vi "Resisitivity of 6-Contact Sample Test.vi"(8 "error in (no error)":errorcluster) -> (0 "error out":errorcluster)   [LabVIEW 2016, in "Hall Effect Library.lvlib"]
doc: "This VI executes the Van Der Pauw Resisitivty Test and returns the voltage measurements V1-V8 taken during the test."
uses:
  Hall Effect Library.lvlib
  Controls/Measurement.ctl
  Public/Controls/Data Items.ctl
  Public/Controls/Tests.ctl
  Global Variables/Test Settings.vi
  Global Variables/Instrument Locations.vi
  Global Variables/Hall Effect Data.vi
panel:
  out "Soak Until":timestamp
  out "Measurement":T1
  out "Test Step":T2(ring)
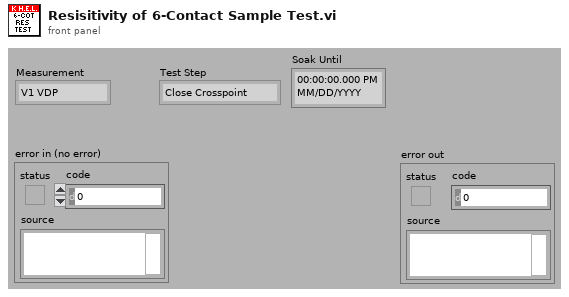
[diagram p1: front panel]
types:
  T1 = typedef "Hall Effect Library.lvlib/Measurement.ctl" = enum16{"V1 VDP", "V2 VDP", "V3 VDP", "V4 VDP", "V5 VDP", "V6 VDP", "V7 VDP", "V8 VDP", "V1 HE", "V2 HE", "V3 HE", "V4 HE", "V5 HE", "V6 HE", "V7 HE", "V8 HE", "V1 Res Bar", "V1 Hall Bar", "V1 Res 6-Cot", "V2 Res 6-Cot", "V3 Res 6-Cot", "V4 Res 6-Cot", "V1 Hall 6-Cot", "V2 Hall 6-Cot", "V3 Hall 6-Cot", "V4 Hall 6-Cot", "V5 Hall 6-Cot", "V6 Hall 6-Cot", "V7 Hall 6-Cot", "V8 Hall 6-Cot", "V1 Res 8-Cot", "V2 Res 8-Cot", "V3 Res 8-Cot", "V4 Res 8-Cot", "V1 Hall 8-Cot", "V2 Hall 8-Cot", "V3 Hall 8-Cot", "V4 Hall 8-Cot"}
  T2 = enum16{"Close Crosspoint", "Soak 1", "Zero Ammeter", "Zero Voltmeter", "I-SRC On", "Init Ammeter", "Soak 2", "Measure I", "Measure V", "I-SRC Off", "Open Crosspoint", "Done"}
  T3 = typedef "Hall Effect Library.lvlib/Resisitivity.ctl" = enum16{"Low", "High"}
  T4 = typedef "Hall Effect Library.lvlib/Tests.ctl" = enum16{"Van Der Pauw", "Hall Effect", "Bar Sample Resistivity", "Bar Sample Hall ", "6-Contact Sample Resistivity", "6-Contact Sample Hall", "8-Contact Sample Resistivity", "8-Contact Sample Hall", ""}
  T5 = typedef "Hall Effect Library.lvlib/Data Items.ctl" = enum16{"V1 Van Der Pauw", "V2 Van Der Pauw", "V3 Van Der Pauw", "V4 Van Der Pauw", "V5 Van Der Pauw", "V6 Van Der Pauw", "V7 Van Der Pauw", "V8 Van Der Pauw", "V1 Hall Effect", "V2 Hall Effect", "V3 Hall Effect", "V4 Hall Effect", "V5 Hall Effect", "V6  Hall Effect", "V7 Hall Effect", "V8 Hall Effect", "V1 Res Bar", "V1 Hall Bar", "V1 Res 6-Cot", "V2 Res 6-Cot", "V3 Res 6-Cot", "V4 Res 6-Cot", "V1 Hall 6-Cot", "V2 Hall 6-Cot", "V3 Hall 6-Cot", "V4 Hall 6-Cot", "V5 Hall 6-Cot", "V6 Hall 6-Cot", "V7 Hall 6-Cot", "V8 Hall 6-Cot", "V1 Res 8-Cot", "V2 Res 8-Cot", "V3 Res 8-Cot", "V4 Res 8-Cot", "V1 Hall 8-Cot", "V2 Hall 8-Cot", "V3 Hall 8-Cot", "V4 Hall 8-Cot", "Van Der Pauw Results", "Hall Effect Results", "Bar Sample Resistivity Results", "Bar Sample Hall Results", "6-Contact Resistivity Results", "6-Contact Hall Results", "8-Contact Resistivity Results", "8-Contact Hall Results"}
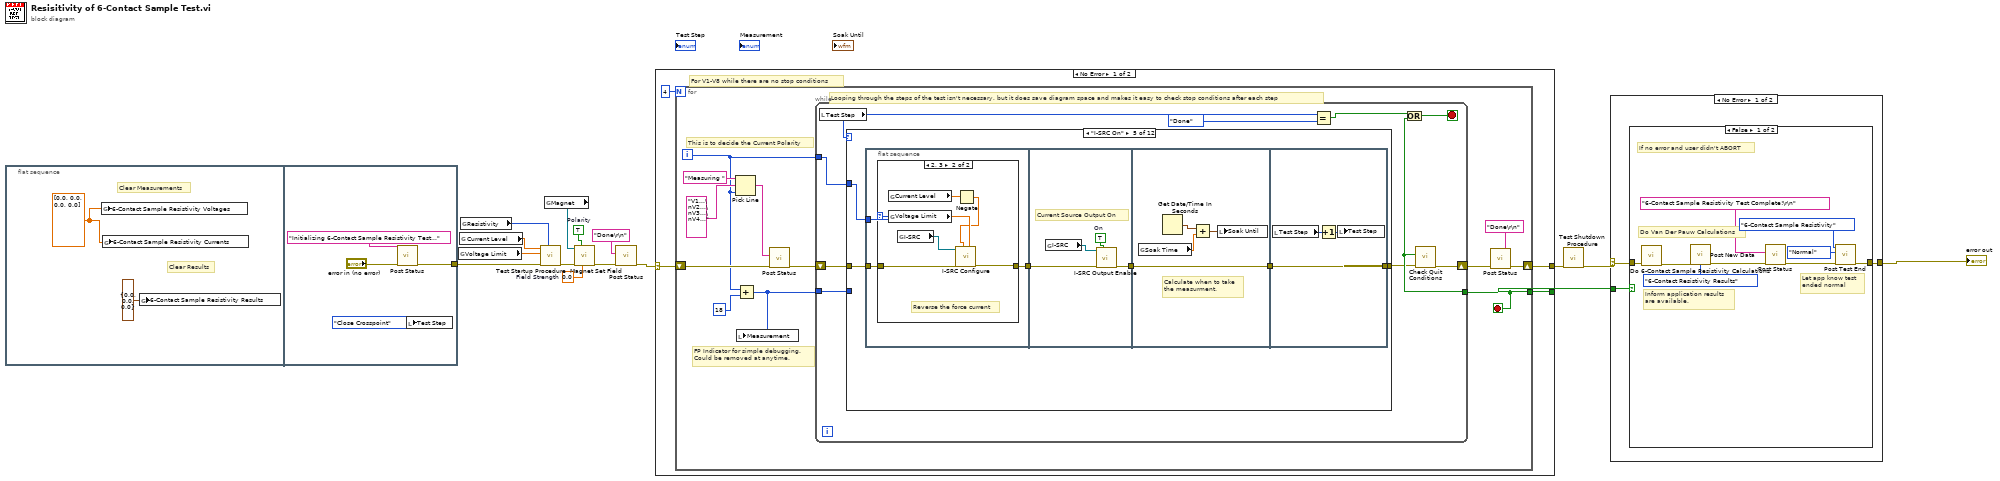
[diagram p0: block diagram]
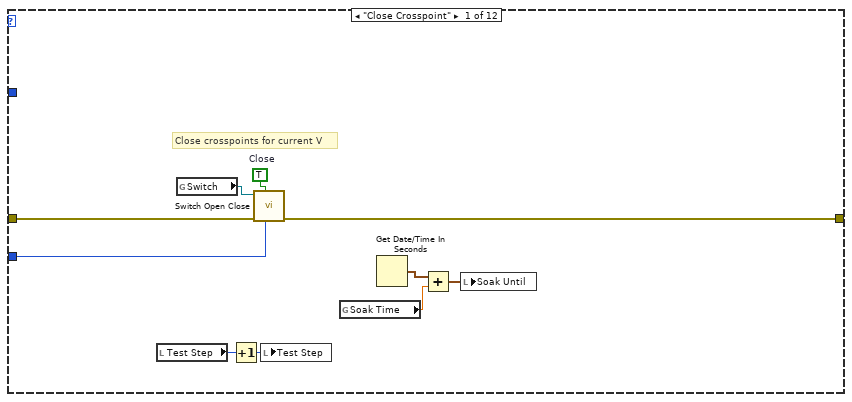
[diagram p2: hidden frame]
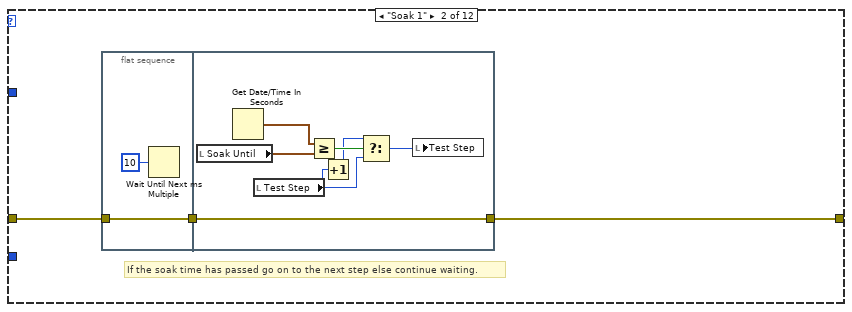
[diagram p3: hidden frame]
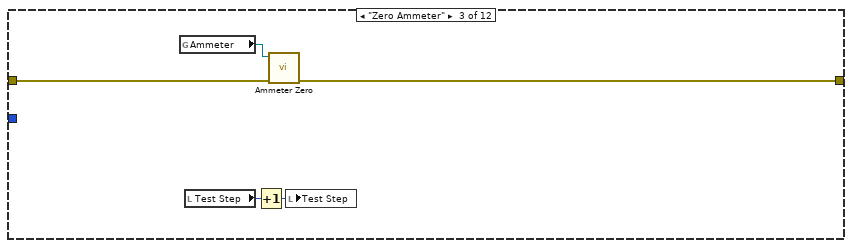
[diagram p4: hidden frame]
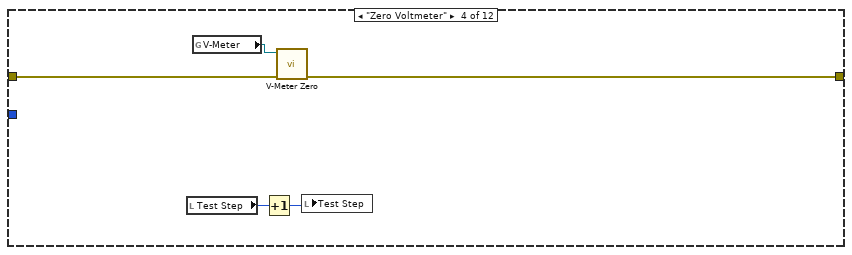
[diagram p5: hidden frame]
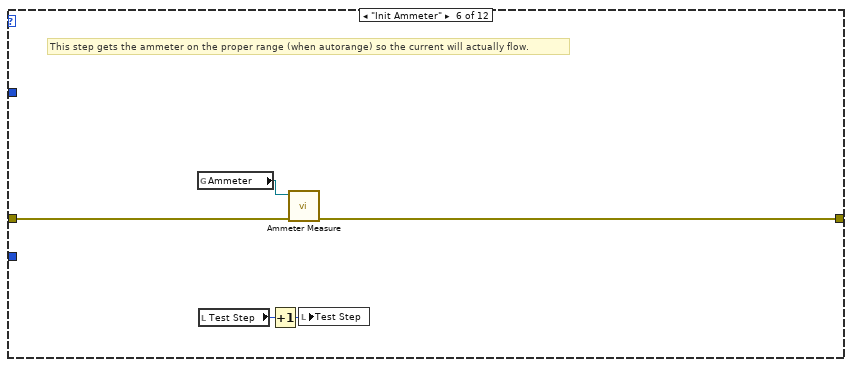
[diagram p7: hidden frame]
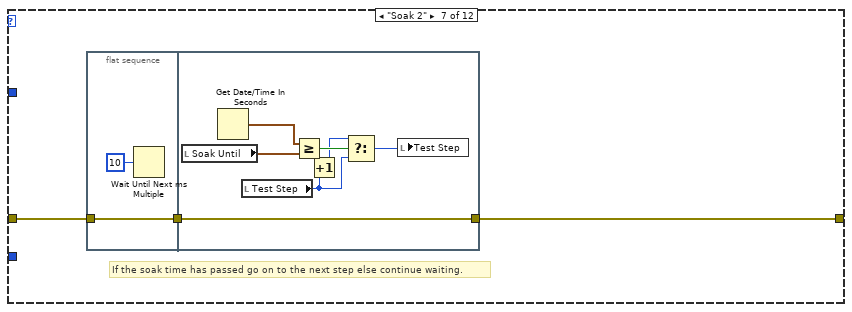
[diagram p8: hidden frame]
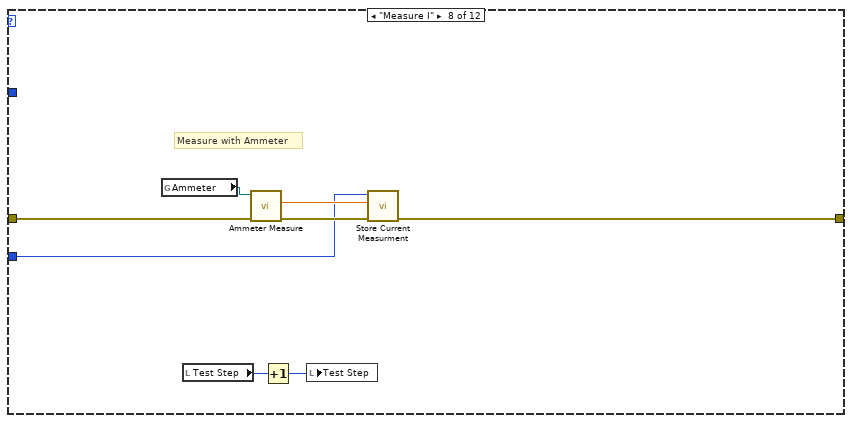
[diagram p9: hidden frame]
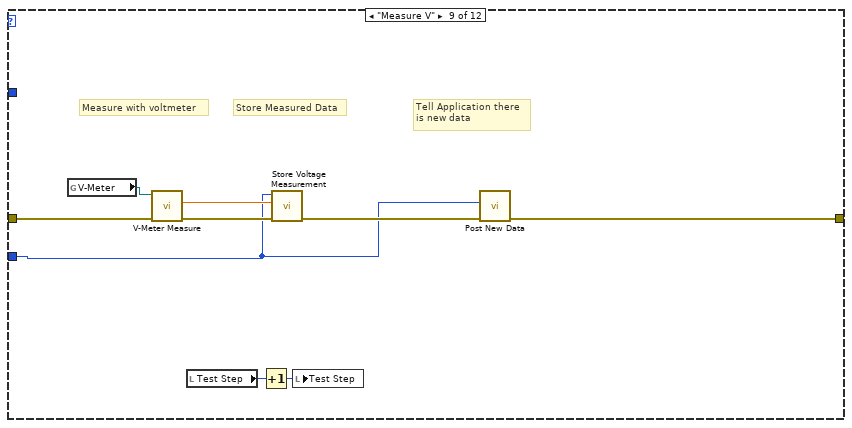
[diagram p10: hidden frame]
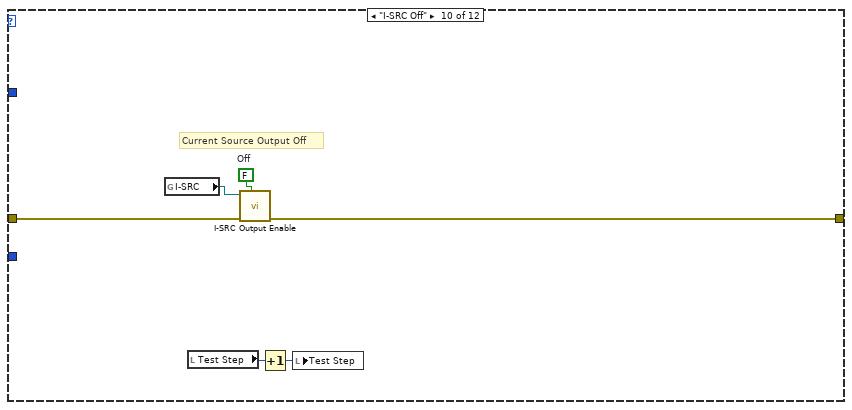
[diagram p11: hidden frame]
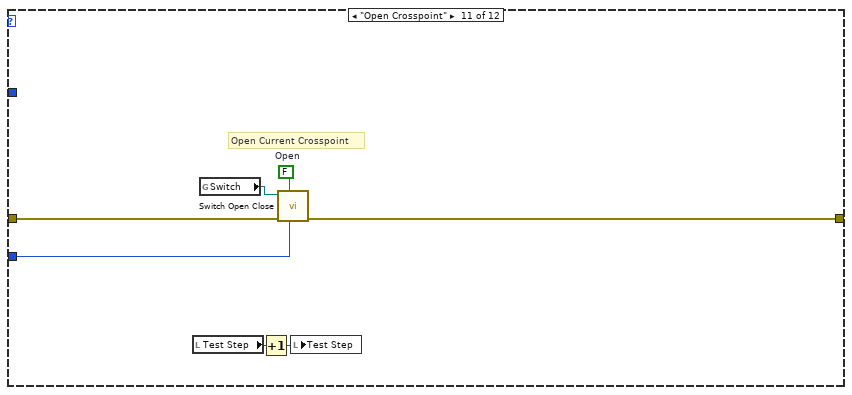
[diagram p12: hidden frame]
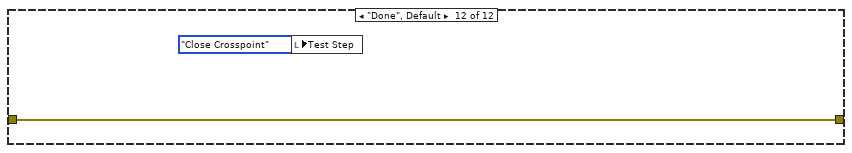
[diagram p13: hidden frame]
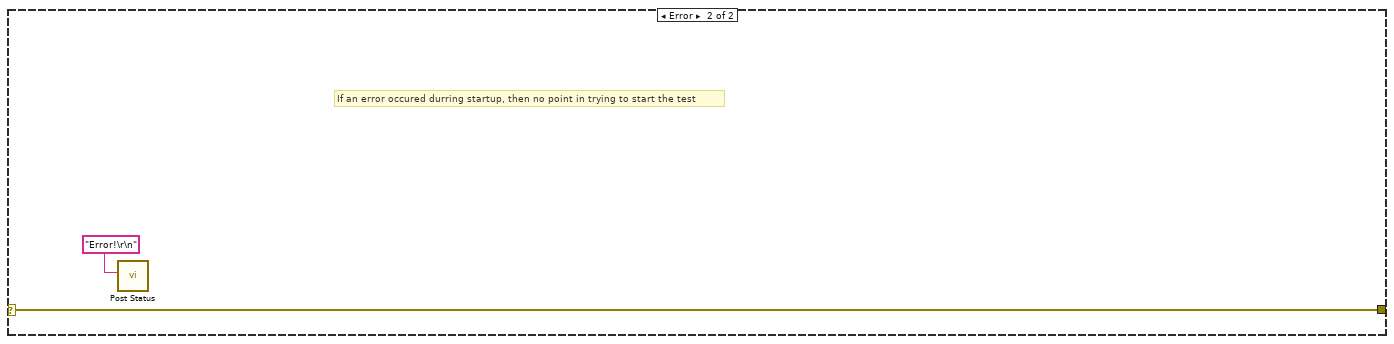
[diagram p14: hidden frame]
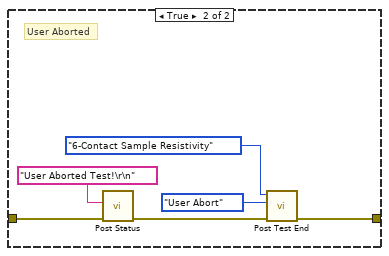
[diagram p15: hidden frame]
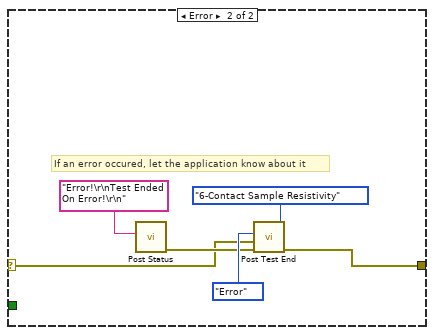
[diagram p16: hidden frame]
diagram:
  w5 = TRUE  # Polarity
  w6 = 0.0  # Field Strength
  n1 = flat-sequence {
    tunnel: [w21] -> w8
    frame #0 {
      w17 = dbl[] [0.0, 0.0, 0.0, 0.0] ("6-Contact Sample Resistivity Voltages")
      # "Clear Results"
      # "Clear Measurements"
      n2 = global write "Hall Effect Data.vi" "6-Contact Sample Resistivity Voltages"(w17) -> ()
      n3 = global write "Hall Effect Data.vi" "6-Contact Sample Resistivity Currents"(w17) -> ()
      n4 = global write "Hall Effect Data.vi" "6-Contact Sample Resistivity Results"(cluster{"PAvg":dbl, "PA":dbl, "PB":dbl} {"PAvg"=0.0, "PA"=0.0, "PB"=0.0} ("6-Contact Sample Resistivity Results")) -> ()
    }
    frame #1 {
      n5 = call "Post Status.vi"("error in (no error)"="error in (no error)", "Status Message"="Initializing 6-Contact Sample Resistivity Test...") -> ("error out"=w21:errorcluster)  [unwired: 9 out]
      n6 = local write "Test Step"(T2."Close Crosspoint" ("Test Step")) -> ()
    }
  }
  n7 = global read "Test Settings.vi" "Voltage Limit"() -> (w9:dbl)
  n8 = global read "Test Settings.vi" "Current Level"() -> (w10:dbl)
  n9 = global read "Test Settings.vi" "Resistivity"() -> (w11:T3)
  n10 = call "Test Startup Procedure.vi"("Resistivity"=w11, "error in (no error)"=w8, "Voltage Limit"=w9, "Current Level"=w10) -> ("error out"=w3:errorcluster)  [unwired: 7 out]
  n11 = global read "Instrument Locations.vi" "Magnet"() -> (w4:refnum<visa-resource-name>)
  n12 = call "Magnet Set Field.vi"("Field Strength"=w6, "Polarity"=w5, "error in (no error)"=w3, "VISA resource name in"=w4) -> ("error out"=w2:errorcluster)  [unwired: 7 out]
  n13 = call "Post Status.vi"("error in (no error)"=w2, "Status Message"="Done\r\n") -> ("error out"=w13:errorcluster)  [unwired: 9 out]
  n14 = case shown="No Error" w13 {
    selector: w13 -> [w23 w157]
    tunnel: [w25 w157] -> w12
    tunnel: [w24 _] -> w14
    frame No Error {
      # "For V1-V8 while there are no stop conditions"
      n15 = for {
        N: 4 -> [_]
        shift-right: [w30] -> w25
        shift-left: w23 -> [w33]
        tunnel: [w29] -> w24
        i -> [w28]
        stop <- w29 stop-if-true
        # "This is to decide the Current Polarity"
        # "FP Indicator for simple debugging.\nCould be removed at anytime."
        # "Looping through the steps of the test isn't necessary, but it does save diagram space and makes it easy to check stop conditions after each step"
        n16 = Pick Line(string ("")="Measuring ", multi-line string="V1...\nV2...\nV3...\nV4...", line index=w28) -> (output string=w35:string)
        n17 = Add(x=w28, y=18) -> (x+y=w27:i32)
        n18 = local write "Measurement"(w27) -> ()
        n19 = call "Post Status.vi"("error in (no error)"=w33, "Status Message"=w35) -> ("error out"=w34:errorcluster)  [unwired: 9 out]
        n20 = while {
          shift-right: [w45] -> w31
          shift-left: w34 -> [w47]
          tunnel: w27 -> [w46]
          tunnel: [w41] -> w29
          tunnel: w28 -> [w38]
          stop <- w44 stop-if-true
          n21 = local read "Test Step"() -> (w42:T2)
          n22 = case shown="\"I-SRC On\"" w42 {
            tunnel: [w55 w58 w72 w77 w84 w110 w113 w128 w135 w143 w151 w155] -> w40
            tunnel: w47 -> [w54 w59 w73 w78 w85 w111 w114 w130 w139 w144 w150 w155]
            tunnel: w46 -> [w53 _ _ _ _ _ _ w126 w132 _ w149 _]
            tunnel: w38 -> [_ _ _ _ w80 _ _ _ _ _ _ _]
            frame "Close Crosspoint" {
              w56 = TRUE  # Close
              # "Close crosspoints for current V"
              n23 = local read "Test Step"() -> (w49:T2)
              n24 = global read "Instrument Locations.vi" "Switch"() -> (w57:refnum<visa-resource-name>)
              n25 = Increment(x=w49) -> (x+1=w48:T2)
              n26 = call "Switch Open Close.vi"("Measurement"=w53, "Open/Close (F: Open)"=w56, "error in (no error)"=w54, "VISA resource name in"=w57) -> ("error out"=w55:errorcluster)  [unwired: 7 out]
              n27 = local write "Test Step"(w48) -> ()
              n28 = global read "Test Settings.vi" "Soak Time"() -> (w51:dbl)
              n29 = Get Date/Time In Seconds() -> (seconds since 1Jan1904=w50:timestamp)
              n30 = Add(x=w50, y=w51) -> (x+y=w52:timestamp)
              n31 = local write "Soak Until"(w52) -> ()
            }
            frame "Soak 1" {
              # "If the soak time has passed go on to the next step else continue waiting."
              n32 = flat-sequence {
                tunnel: w59 -> [w61]
                tunnel: [w61] -> w60
                tunnel: [w65] -> w58
                tunnel: w60 -> [w65]
                frame #0 {
                  n33 = Wait Until Next ms Multiple(millisecond multiple=u32 10) -> ()  [unwired: 1 out]
                }
                frame #1 {
                  n34 = local read "Soak Until"() -> (w68:timestamp)
                  n35 = Get Date/Time In Seconds() -> (seconds since 1Jan1904=w69:timestamp)
                  n36 = local read "Test Step"() -> (w64:T2)
                  n37 = Greater Or Equal?(x=w69, y=w68) -> (x >= y?=w67:bool)
                  n38 = Increment(x=w64) -> (x+1=w63:T2)
                  n39 = Select(t=w63, s=w67, f=w64) -> (s? t:f=w66:T2)
                  n40 = local write "Test Step"(w66) -> ()
                }
              }
            }
            frame "Zero Ammeter" {
              n41 = global read "Instrument Locations.vi" "Ammeter"() -> (w74:refnum<visa-resource-name>)
              n42 = local read "Test Step"() -> (w71:T2)
              n43 = Increment(x=w71) -> (x+1=w70:T2)
              n44 = call "Ammeter Zero.vi"("error in (no error)"=w73, "VISA resource name in"=w74) -> ("error out"=w72:errorcluster)  [unwired: 9 out]
              n45 = local write "Test Step"(w70) -> ()
            }
            frame "Zero Voltmeter" {
              n46 = local read "Test Step"() -> (w75:T2)
              n47 = global read "Instrument Locations.vi" "V-Meter"() -> (w79:refnum<visa-resource-name>)
              n48 = Increment(x=w75) -> (x+1=w76:T2)
              n49 = call "V-Meter Zero.vi"("error in (no error)"=w78, "VISA resource name in"=w79) -> ("error out"=w77:errorcluster)  [unwired: 9 out]
              n50 = local write "Test Step"(w76) -> ()
            }
            frame "I-SRC On" {
              n51 = flat-sequence {
                tunnel: w85 -> [w87]
                tunnel: [w86] -> w81
                tunnel: w80 -> [w88]
                tunnel: [w96] -> w83
                tunnel: w81 -> [w97]
                tunnel: w83 -> [w103]
                tunnel: [w103] -> w82
                tunnel: [w106] -> w84
                tunnel: w82 -> [w106]
                frame #0 {
                  n52 = case shown="2, 3" w88 {
                    tunnel: w87 -> [w89 w93]
                    tunnel: [w89 w92] -> w86
                    frame 0, 1, Default {
                    }
                    frame 2, 3 {
                      # "Reverse the force current"
                      n53 = global read "Test Settings.vi" "Current Level"() -> (w91:dbl)
                      n54 = global read "Test Settings.vi" "Voltage Limit"() -> (w94:dbl)
                      n55 = global read "Instrument Locations.vi" "I-SRC"() -> (w95:refnum<visa-resource-name>)
                      n56 = Negate(x=w91) -> (-x=w90:dbl)
                      n57 = call "I-SRC Configure.vi"("Voltage Limit"=w94, "Current Level"=w90, "error in (no error)"=w93, "VISA resource name in"=w95) -> ("error out"=w92:errorcluster)  [unwired: 6 in, 1 out]
                    }
                  }
                }
                frame #1 {
                  w98 = TRUE  # On
                  # "Current Source Output On"
                  n58 = global read "Instrument Locations.vi" "I-SRC"() -> (w99:refnum<visa-resource-name>)
                  n59 = call "I-SRC Output Enable.vi"("Output (Off)"=w98, "error in (no error)"=w97, "VISA resource name in"=w99) -> ("error out"=w96:errorcluster)  [unwired: 8 out]
                }
                frame #2 {
                  # "Calculate when to take\nthe measurment."
                  n60 = global read "Test Settings.vi" "Soak Time"() -> (w101:dbl)
                  n61 = Get Date/Time In Seconds() -> (seconds since 1Jan1904=w100:timestamp)
                  n62 = Add(x=w100, y=w101) -> (x+y=w102:timestamp)
                  n63 = local write "Soak Until"(w102) -> ()
                }
                frame #3 {
                  n64 = local read "Test Step"() -> (w105:T2)
                  n65 = Increment(x=w105) -> (x+1=w104:T2)
                  n66 = local write "Test Step"(w104) -> ()
                }
              }
            }
            frame "Init Ammeter" {
              # "This step gets the ammeter on the proper range (when autorange) so the current will actually flow."
              n67 = global read "Instrument Locations.vi" "Ammeter"() -> (w109:refnum<visa-resource-name>)
              n68 = local read "Test Step"() -> (w108:T2)
              n69 = Increment(x=w108) -> (x+1=w107:T2)
              n70 = call "Ammeter Measure.vi"("error in (no error)"=w111, "VISA resource name in"=w109) -> ("error out"=w110:errorcluster)  [unwired: 9 out]
              n71 = local write "Test Step"(w107) -> ()
            }
            frame "Soak 2" {
              # "If the soak time has passed go on to the next step else continue waiting."
              n72 = flat-sequence {
                tunnel: w114 -> [w115]
                tunnel: [w115] -> w112
                tunnel: [w119] -> w113
                tunnel: w112 -> [w119]
                frame #0 {
                  n73 = Wait Until Next ms Multiple(millisecond multiple=u32 10) -> ()  [unwired: 1 out]
                }
                frame #1 {
                  n74 = local read "Soak Until"() -> (w122:timestamp)
                  n75 = Get Date/Time In Seconds() -> (seconds since 1Jan1904=w123:timestamp)
                  n76 = local read "Test Step"() -> (w117:T2)
                  n77 = Greater Or Equal?(x=w123, y=w122) -> (x >= y?=w121:bool)
                  n78 = Increment(x=w117) -> (x+1=w118:T2)
                  n79 = Select(t=w118, s=w121, f=w117) -> (s? t:f=w120:T2)
                  n80 = local write "Test Step"(w120) -> ()
                }
              }
            }
            frame "Measure I" {
              # "Measure with Ammeter"
              n81 = global read "Instrument Locations.vi" "Ammeter"() -> (w131:refnum<visa-resource-name>)
              n82 = local read "Test Step"() -> (w125:T2)
              n83 = call "Ammeter Measure.vi"("error in (no error)"=w130, "VISA resource name in"=w131) -> ("error out"=w129:errorcluster, "Measurement"=w127:dbl)  [unwired: 8 out]
              n84 = Increment(x=w125) -> (x+1=w124:T2)
              n85 = local write "Test Step"(w124) -> ()
              n86 = call "Store Current Measurment.vi"("error in"=w129, "Value"=w127, "Measurement"=w126) -> ("error out"=w128:errorcluster)  [unwired: 8 out]
            }
            frame "Measure V" {
              # "Tell Application there\nis new data"
              # "Store Measured Data"
              # "Measure with voltmeter"
              n87 = global read "Instrument Locations.vi" "V-Meter"() -> (w140:refnum<visa-resource-name>)
              n88 = call "V-Meter Measure.vi"("error in (no error)"=w139, "VISA resource name in"=w140) -> ("error out"=w138:errorcluster, "Measurement"=w137:dbl)  [unwired: 1 in, 7 out]
              n89 = local read "Test Step"() -> (w134:T2)
              n90 = Increment(x=w134) -> (x+1=w133:T2)
              n91 = call "Store Voltage Measurement.vi"("error in"=w138, "Value"=w137, "Measurement"=w132) -> ("error out"=w136:errorcluster)  [unwired: 8 out]
              n92 = local write "Test Step"(w133) -> ()
              n93 = call "Post New Data.vi"("error in (no error)"=w136, "Data Item"=w132) -> ("error out"=w135:errorcluster)  [unwired: 9 out]
            }
            frame "I-SRC Off" {
              w145 = FALSE  # Off
              # "Current Source Output Off"
              n94 = global read "Instrument Locations.vi" "I-SRC"() -> (w146:refnum<visa-resource-name>)
              n95 = local read "Test Step"() -> (w142:T2)
              n96 = call "I-SRC Output Enable.vi"("Output (Off)"=w145, "error in (no error)"=w144, "VISA resource name in"=w146) -> ("error out"=w143:errorcluster)  [unwired: 8 out]
              n97 = Increment(x=w142) -> (x+1=w141:T2)
              n98 = local write "Test Step"(w141) -> ()
            }
            frame "Open Crosspoint" {
              w152 = FALSE  # Open
              # "Open Current Crosspoint"
              n99 = local read "Test Step"() -> (w147:T2)
              n100 = global read "Instrument Locations.vi" "Switch"() -> (w153:refnum<visa-resource-name>)
              n101 = Increment(x=w147) -> (x+1=w148:T2)
              n102 = call "Switch Open Close.vi"("Measurement"=w149, "Open/Close (F: Open)"=w152, "error in (no error)"=w150, "VISA resource name in"=w153) -> ("error out"=w151:errorcluster)  [unwired: 7 out]
              n103 = local write "Test Step"(w148) -> ()
            }
            frame "Done", Default {
              n104 = local write "Test Step"(T2."Close Crosspoint" ("Test Step")) -> ()
            }
          }
          n105 = Equal?(x=w42, y=T2."Done") -> (x = y?=w43:bool)
          n106 = call "Check Quit Conditions.vi"("error in (no error)"=w40) -> ("error out"=w45:errorcluster, "Quit?"=w41:bool)  [unwired: 9 out]
          n107 = Or(x=w43, y=w41) -> (x .or. y?=w44:bool)
        }
        n108 = call "Post Status.vi"("error in (no error)"=w31, "Status Message"="Done\r\n") -> ("error out"=w30:errorcluster)  [unwired: 9 out]
      }
    }
    frame Error {
      # "If an error occured durring startup, then no point in trying to start the test"
      n109 = call "Post Status.vi"("Status Message"="Error!\r\n") -> ()  [unwired: 1 in, 10 out]
    }
  }
  n110 = call "Test Shutdown Procedure.vi"("error in (no error)"=w12) -> ("error out"=w1:errorcluster)  [unwired: 10 out]
  n111 = case shown="No Error" w1 {
    selector: w1 -> [w159 w177]
    tunnel: w14 -> [w160 _]
    tunnel: [w158 w179] -> w15
    frame No Error {
      n112 = case shown="False" w160 {
        tunnel: w159 -> [w162 w174]
        tunnel: [w165 w171] -> w158
        frame False {
          # "Let app know test\nended normal"
          # "Inform application results\nare available."
          # "Do Van Der Pauw Calculations"
          # "If no error and user didn't ABORT"
          n113 = call "Do 6-Contact Sample Resistivity Calculations.vi"("error in (no error)"=w162) -> ("error out"=w161:errorcluster)  [unwired: 10 in]
          n114 = call "Post New Data.vi"("error in (no error)"=w161, "Data Item"=Data_Items."6-Contact Resistivity Results") -> ("error out"=w167:errorcluster)  [unwired: 9 out]
          n115 = call "Post Status.vi"("error in (no error)"=w167, "Status Message"="6-Contact Sample Resistivity Test Complete!\r\n") -> ("error out"=w164:errorcluster)  [unwired: 9 out]
          n116 = call "Post Test End.vi"("error in (no error)"=w164, "Test End"=enum16{"Normal", "User Abort", "Error"}."Normal", "Test"=Tests."6-Contact Sample Resistivity") -> ("error out"=w165:errorcluster)  [unwired: 1 in, 7 out]
        }
        frame True {
          # "User Aborted"
          n117 = call "Post Status.vi"("error in (no error)"=w174, "Status Message"="User Aborted Test!\r\n") -> ("error out"=w173:errorcluster)  [unwired: 9 out]
          n118 = call "Post Test End.vi"("error in (no error)"=w173, "Test End"=enum16{"Normal", "User Abort", "Error"}."User Abort", "Test"=Tests."6-Contact Sample Resistivity") -> ("error out"=w171:errorcluster)  [unwired: 1 in, 7 out]
        }
      }
    }
    frame Error {
      # "If an error occured, let the application know about it"
      n119 = call "Post Status.vi"("Status Message"="Error!\r\nTest Ended On Error!\r\n") -> ("error out"=w178:errorcluster)  [unwired: 1 in, 9 out]
      n120 = call "Post Test End.vi"("error in (no error)"=w178, "Test End Error (no error)"=w177, "Test End"=enum16{"Normal", "User Abort", "Error"}."Error", "Test"=Tests."6-Contact Sample Resistivity") -> ("error out"=w179:errorcluster)  [unwired: 7 out]
    }
  }
  "error out" <- w15
